vi "Module Cleanup.vi"(8 "error in (no error)":errorcluster, 11 "Log Preparer Module in":refnum<class "Log Preparer Module.lvclass">) -> (0 "error out":errorcluster, 3 "Log Preparer Module out":refnum<class "Log Preparer Module.lvclass">)   [LabVIEW 2020, in "VolatusData.lvlib" / "Log Preparer Module.lvclass"]
uses:
  Log Preparer Module.lvclass
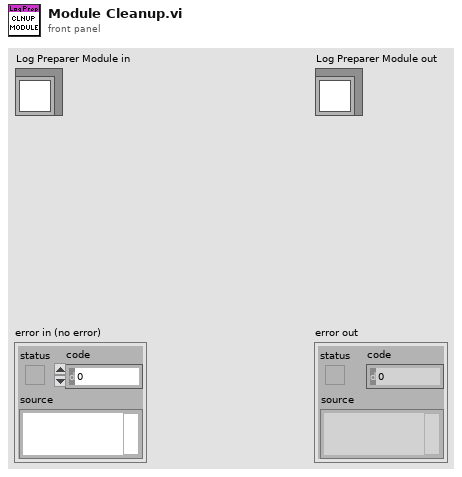
[diagram p1: front panel]
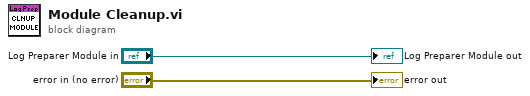
[diagram p0: block diagram]
diagram:
  "error out" <- "error in (no error)"
  "Log Preparer Module out" <- "Log Preparer Module in"
